vi "debugBytes.vi"(7 "outgoing?":bool, 8 "error in (no error)":errorcluster, 10 "Bytes":u8[](array[numeric]) format="%08b", 11 "Connection in":refnum<class "Connection.lvclass">) -> (0 "error out":errorcluster, 3 "Connection out":refnum<class "Connection.lvclass">)   [LabVIEW 2013, in "Connection_GOSPL.lvlib" / "Connection.lvclass"]
uses:
  Connection.lvclass
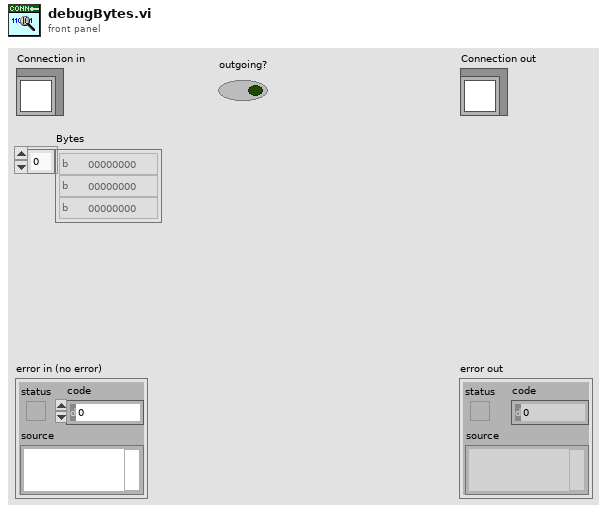
[diagram p1: front panel]
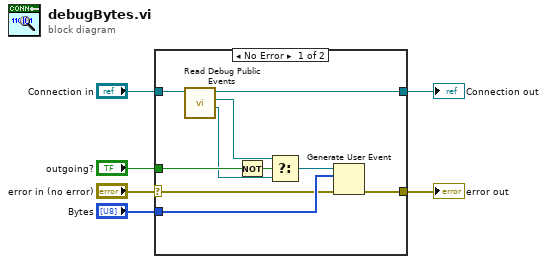
[diagram p0: block diagram]
diagram:
  n1 = case shown="No Error" "error in (no error)" {
    selector: "error in (no error)" -> [w8 w18]
    tunnel: [w7 w18] -> w5
    tunnel: [w15 w17] -> w3
    tunnel: "Connection in" -> [w16 w17]
    tunnel: "outgoing?" -> [w14 _]
    tunnel: "Bytes" -> [w9 _]
    frame No Error {
      n2 = call "Read Debug Public Events.vi"("Connection in"=w16) -> ("outgoing"=w12:refnum<user-event>, "incoming"=w13:refnum<user-event>, "Connection out"=w15:refnum<class "Connection.lvclass">)  [unwired: 7 in, 1 out]
      n3 = Not(x=w14) -> (.not. x?=w10:bool)
      n4 = Select(t=w13, s=w10, f=w12) -> (s? t:f=w11:refnum<user-event>)
      n5 = Generate User Event(user event=w11, event data cluster=w9, error in=w8) -> (error out=w7:errorcluster)  [unwired: 1 in, 1 out]
    }
    frame Error {
    }
  }
  "error out" <- w5
  "Connection out" <- w3
